vi "LEBITVacuum.CreateDBArray.vi"(0 "connection in":refnum<k7>, 2 "query results":string[][](array[string]), 5 "error in":errorcluster, 8 "Associated Panels":string[](array[string])) -> (14 "connection out":refnum<k7>, 16 "DBArray":string[][](array[string]), 17 "Safety Array":string[][](array[string]), 18 "Ambient Measurements":string[][](array[string]), 19 "error out":errorcluster)   [LabVIEW 2014, in "LEBITVacuum.lvlib"]
uses:
  LEBITVacuum.lvlib
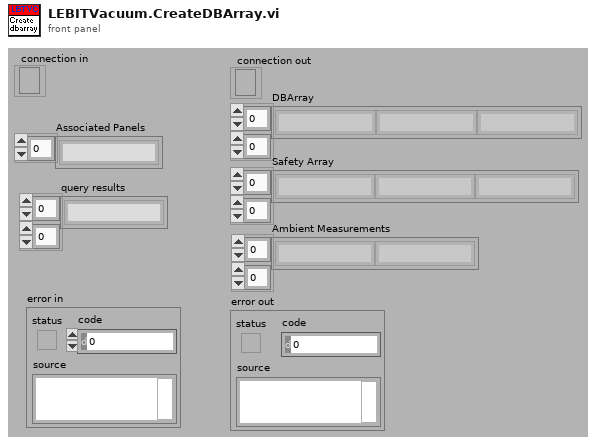
[diagram p1: front panel]
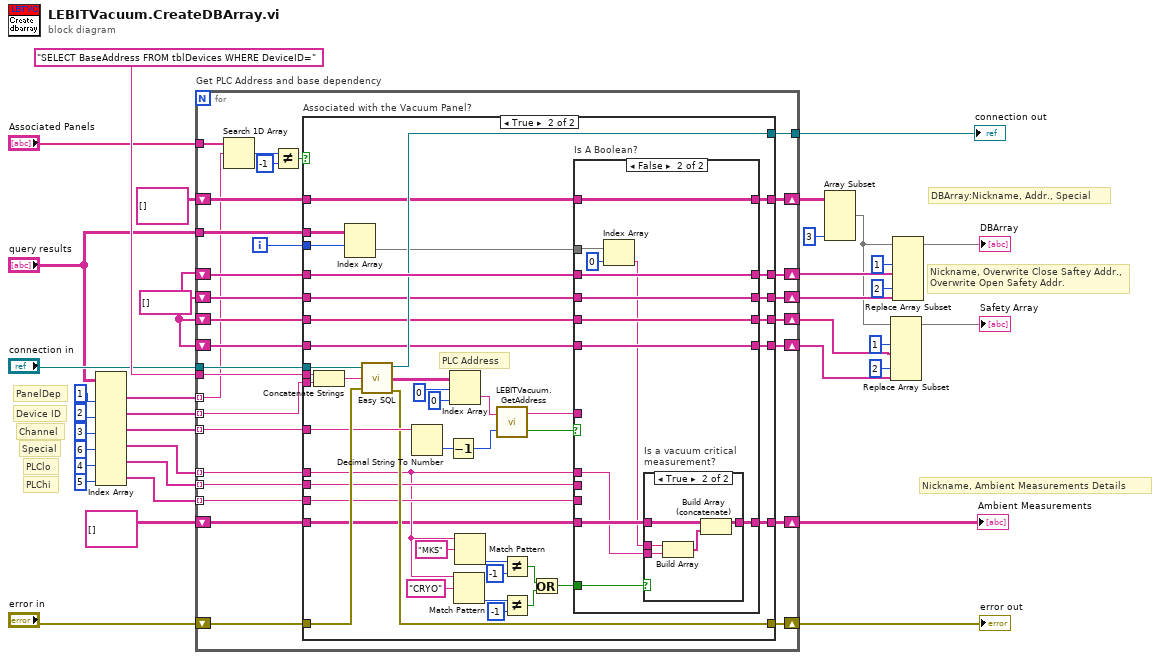
[diagram p0: block diagram]
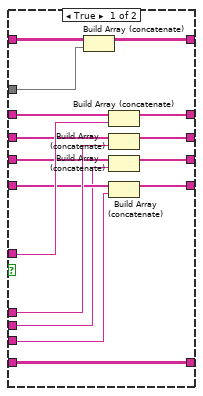
[diagram p3: hidden frame]
diagram:
  w14 = string[] []
  # "PLChi"
  # "PLClo"
  # "Special"
  # "Channel"
  # "PanelDep"
  # "Device ID"
  # "Nickname, Ambient Measurements Details"
  # "Nickname, Overwrite Close Saftey Addr.,\nOverwrite Open Safety Addr."
  # "DBArray:Nickname, Addr., Special"
  n1 = Index Array(array="query results", index (col) #1=1 ("index (row)"), index (col) #2=2 ("disabled index (col)"), index (col) #3=3 ("index (col)"), index (col) #4=6 ("index (col)"), index (col) #5=4 ("index (col)"), index (col) #6=5 ("index (col)")) -> (element #1=w5:string[], element #2=w27:string[], element #3=w30:string[], element #4=w20:string[], element #5=w16:string[], element #6=w15:string[])  [unwired: 6 in]
  n2 = for "Get PLC Address and base dependency" {
    tunnel: w27 -> [w62] mode=indexing
    tunnel: "connection in" -> [w65]
    tunnel: w30 -> [w61] mode=indexing
    shift-right: [w60] -> w33
    shift-left: "error in" -> [w64]
    tunnel: "SELECT BaseAddress FROM tblDevices WHERE DeviceID=" -> [w63]
    shift-right: [w58] -> w36
    shift-left: w14 -> [w59]
    tunnel: [w57] -> w25
    tunnel: "query results" -> [w56]
    shift-right: [w54] -> w22
    shift-left: string[][] [] -> [w55]
    tunnel: w20 -> [w53] mode=indexing
    shift-right: [w51] -> w13
    shift-left: w14 -> [w52]
    tunnel: w16 -> [w49] mode=indexing
    tunnel: w15 -> [w48] mode=indexing
    shift-right: [w44] -> w10
    shift-left: w14 -> [w47]
    shift-right: [w45] -> w9
    shift-left: w14 -> [w46]
    tunnel: w5 -> [w38] mode=indexing
    shift-right: [w42] -> w3
    shift-left: string[][] [] -> [w43]
    tunnel: "Associated Panels" -> [w37]
    i -> [w50]
    n3 = Search 1D Array(1D array=w37, element=w38) -> (index of element=w41:i32)  [unwired: 1 in]
    n4 = Not Equal?(x=w41, y=-1) -> (x != y?=w39:bool)
    n5 = case "Associated with the Vacuum Panel?" shown="True" w39 {
      tunnel: w65 -> [w67 w116]
      tunnel: w64 -> [w68 w115]
      tunnel: w63 -> [_ w114]
      tunnel: w62 -> [_ w113]
      tunnel: w61 -> [_ w110]
      tunnel: [w68 w109] -> w60
      tunnel: w59 -> [w72 w108]
      tunnel: [w72 w107] -> w58
      tunnel: [w67 w99] -> w57
      tunnel: w56 -> [_ w98]
      tunnel: w55 -> [w73 w97]
      tunnel: [w73 w96] -> w54
      tunnel: w53 -> [_ w85]
      tunnel: w52 -> [w71 w94]
      tunnel: [w71 w93] -> w51
      tunnel: w50 -> [_ w92]
      tunnel: w49 -> [_ w91]
      tunnel: w48 -> [_ w90]
      tunnel: w47 -> [w70 w89]
      tunnel: w46 -> [w69 w88]
      tunnel: [w69 w87] -> w45
      tunnel: [w70 w86] -> w44
      tunnel: w43 -> [w66 w75]
      tunnel: [w66 w74] -> w42
      frame False {
      }
      frame True {
        # "PLC Address"
        n6 = Concatenate Strings(w114, w113) -> (w112:string)
        n7 = Index Array(array=w98, index (row)=w92) -> (element=w95:string[])  [unwired: 1 in]
        n8 = call <vilib>:"Easy SQL.vi"("connection"=w116, "SQL statement"=w112, "error in (no error)"=w115) -> ("connection"=w99:refnum<k7>, "error out"=w109:errorcluster, "query results"=w111:string[][])  [unwired: 2 out]
        n9 = Decimal String To Number(string=w110) -> (number=w105:i32)  [unwired: 2 in, 1 out]
        n10 = Decrement(x=w105) -> (x-1=w103:i32)
        n11 = Index Array(array=w111, index (row)=0, index (col)=0 ("disabled index (col)")) -> (element=w102:string)
        n12 = Match Pattern(string=w85, regular expression="CRYO") -> (offset past match=w81:i32)  [unwired: 1 in, 3 out]
        n13 = Match Pattern(string=w85, regular expression="MKS") -> (offset past match=w82:i32)  [unwired: 1 in, 3 out]
        n14 = call "LEBITVacuum.GetAddress.vi"("channel# (dec)"=w103, "base Actual addr. (oct)"=w102) -> ("is a boolean?"=w100:bool, "act. addr. (oct)"=w101:string)
        n15 = Not Equal?(x=w82, y=-1) -> (x != y?=w77:bool)
        n16 = Not Equal?(x=w81, y=-1) -> (x != y?=w78:bool)
        n17 = Or(x=w77, y=w78) -> (x .or. y?=w76:bool)
        n18 = case "Is A Boolean?" shown="False" w100 {
          tunnel: w108 -> [w132 w143]
          tunnel: [w131 w143] -> w107
          tunnel: w101 -> [w130 _]
          tunnel: w97 -> [w129 w144]
          tunnel: [w128 w144] -> w96
          tunnel: w95 -> [w127 w135]
          tunnel: w85 -> [w124 w136]
          tunnel: w94 -> [w126 w142]
          tunnel: [w125 w142] -> w93
          tunnel: w91 -> [w119 _]
          tunnel: w90 -> [w118 _]
          tunnel: w89 -> [w123 w141]
          tunnel: w88 -> [w122 w140]
          tunnel: [w121 w140] -> w87
          tunnel: [w120 w141] -> w86
          tunnel: w76 -> [_ w139]
          tunnel: w75 -> [w117 w138]
          tunnel: [w117 w137] -> w74
          frame True {
            n19 = Build Array (concatenate)(w129, w127) -> (w128:string[][])
            n20 = Build Array (concatenate)(w132, w130) -> (w131:string[])
            n21 = Build Array (concatenate)(w126, w124) -> (w125:string[])
            n22 = Build Array (concatenate)(w123, w119) -> (w120:string[])
            n23 = Build Array (concatenate)(w122, w118) -> (w121:string[])
          }
          frame False {
            n24 = Index Array(array=w135, index=0) -> (element=w133:string)
            n25 = case "Is a vacuum critical\nmeasurement?" shown="True" w139 {
              tunnel: w138 -> [w145 w150]
              tunnel: [w145 w149] -> w137
              tunnel: w136 -> [_ w148]
              tunnel: w133 -> [_ w146]
              frame False {
              }
              frame True {
                n26 = Build Array(w146, w148) -> (w147:string[])
                n27 = Build Array (concatenate)(w150, w147) -> (w149:string[][])
              }
            }
          }
        }
      }
    }
  }
  "error out" <- w33
  "connection out" <- w25
  "Ambient Measurements" <- w3
  n28 = Array Subset(array=w22, length (col)=3 ("length")) -> (w11:string[][])  [unwired: 3 in]
  n29 = Replace Array Subset(array=w11, new element #1=w10, index (col) #1=1 ("disabled index (col)"), new element #2=w9, index (col) #2=2 ("disabled index (col)")) -> (→"Safety Array":string[][])  [unwired: 2 in]
  n30 = Replace Array Subset(array=w11, new element #1=w36, index (col) #1=1 ("disabled index (col)"), new element #2=w13, index (col) #2=2 ("index (col)")) -> (→"DBArray":string[][])  [unwired: 2 in]
